vi "PSU_Output.vi"(8 "error in (no error)":errorcluster, 10 "Output %":dbl, 11 "DataCluster in":T1={"Core"={"Current VI Reference"=refnum, "Close Panel on Exit?"=FALSE, "Exit"=FALSE}, "Connections"={"cDAQ Therm"={"Task"="", "Connected"=FALSE, "Active"=FALSE}, "cDAQ Voltage"={"Task"="", "Connected"=FALSE, "Active"=FALSE}, "cDAQ ID"="", "Camera"={"Session"="", "Connected"=FALSE, "Active"=FALSE}, "PSU"={"Port"="", "Connected"=FALSE, "Active"=FALSE}}, "Data Acquisition"={"Setup"={"Label"="", "Operator"="", "Notes"="", "TempGrad"=1.0, "TargetTemp"=1.0, "Sample Volume"=1.0}, "Camera"={"Image"=refnum, "Save Image"=refnum, "Image Frequency"=20, "Rectangle"={"Left"=0, "Top"=0, "Right"=0, "Bottom"=0, "Rotation"=0.0}}, "Thermistor"={"Sample Size"=1, "Calibration"={"B0.100"=[], "R25"=[], "c"=[], "State"=[], "V_S"=5.0, "R_S"=100.0}, "Timing Mode"=14713}, "Partition"={"Data"=[], "Cell Label"="", "Cell Color"=0, "Height"=10, "Width"=16, "Grid"=[]}, "Queue"={"Queue"=refnum, "Size"=1}, "Sample Rate"=20, "Active"=FALSE, "Ready"=FALSE, "Graph Mode"=0}, "Control"={"Sample Rate"=1, "PID gains"={"proportional gain (Kc)"=1.0, "integral time (Ti, min)"=0.01, "derivative time (Td, min)"=0.0}}} {"Control"."PID gains"."derivative time (Td, min)" format="%.3f"; "Control"."PID gains"."integral time (Ti, min)" format="%.3f"; "Control"."PID gains"."proportional gain (Kc)" format="%.3f"; "Control"."Sample Rate" min=1 max=20 step=1 format="%.0f Samples/sec"; "Data Acquisition"."Graph Mode" items=["Average Temperature", "Individual Temperatures"]; "Data Acquisition"."Thermistor"."Timing Mode" items=["Automatic"=16097, "High Resolution"=10195, "High Speed"=14712, "Best 50 Hz Rejection"=14713, "Best 60 Hz Rejection"=14714, "Custom"=10137]; "Data Acquisition"."Thermistor"."Calibration"."R_S" min=0.1 max=1000.0 format="%#_g kOhm"; "Data Acquisition"."Thermistor"."Calibration"."V_S" min=5.0 max=48.0 format="%#_g V"; "Data Acquisition"."Thermistor"."Calibration"."R25" min=0.1 max=1000.0 format="%#_g kOhm"; "Data Acquisition"."Thermistor"."Calibration"."B0.100" min=100.0 max=10000.0 format="%#_g K"; "Data Acquisition"."Thermistor"."Sample Size" min=1 max=200; "Data Acquisition"."Sample Rate" min=20 max=240 format="%.0f samples/min"; "Data Acquisition"."Queue"."Size" min=1 max=200; "Data Acquisition"."Camera"."Rectangle"."Rotation" min=-90.0 max=90.0 step=1.0 format="%.2f"; "Data Acquisition"."Camera"."Rectangle"."Left" scale=0.0..1024.0; "Data Acquisition"."Camera"."Rectangle"."Right" scale=0.0..1024.0; "Data Acquisition"."Camera"."Image Frequency" min=1 max=60 step=1; "Data Acquisition"."Setup"."Sample Volume" min=0.0 max=500.0 format="%#_g µL"; "Data Acquisition"."Setup"."TargetTemp" min=-40.0 max=40.0 step=0.5 format="%#_g °C"; "Data Acquisition"."Setup"."TempGrad" min=-100.0 max=100.0 step=0.1 format="%#_g °C/min"}) -> (0 "error out":errorcluster, 1 "valid?":bool, 2 "Output % duplicate":dbl)   [LabVIEW 2020]
uses:
  DataCluster.ctl
  <vilib>/userDefined/High Color/IMAQdx.ctl
  <vilib>/vision/Image Controls.llb/IMAQ Image.ctl
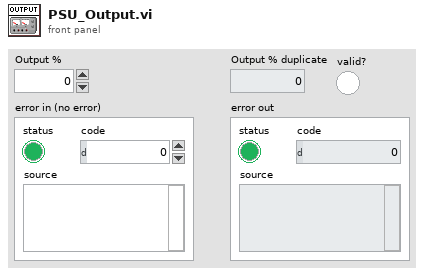
[diagram p1: front panel]
types:
  T1 = typedef "DataCluster.ctl" = cluster{"Core":cluster{"Current VI Reference":refnum<vi>, "Close Panel on Exit?":bool, "Exit":bool}, "Connections":cluster{"cDAQ Therm":cluster{"Task":refnum<k21>, "Connected":bool, "Active":bool}, "cDAQ Voltage":cluster{"Task":refnum<k21>, "Connected":bool, "Active":bool}, "cDAQ ID":string, "Camera":cluster{"Session":T2, "Connected":bool, "Active":bool}, "PSU":cluster{"Port":refnum<visa-resource-name>, "Connected":bool, "Active":bool}}, "Data Acquisition":cluster{"Setup":cluster{"Label":string, "Operator":string, "Notes":string, "TempGrad":dbl, "TargetTemp":dbl, "Sample Volume":dbl}, "Camera":cluster{"Image":T3, "Save Image":T3, "Image Frequency":i32, "Rectangle":T4}, "Thermistor":cluster{"Sample Size":i32, "Calibration":cluster{"B0.100":dbl[], "R25":dbl[], "c":dbl[][], "State":bool[], "V_S":dbl, "R_S":dbl}, "Timing Mode":i32}, "Partition":cluster{"Data":string[][], "Cell Label":string, "Cell Color":u32, "Height":i32, "Width":i32, "Grid":string[][]}, "Queue":cluster{"Queue":refnum<queue>, "Size":i32}, "Sample Rate":i32, "Active":bool, "Ready":bool, "Graph Mode":u16}, "Control":cluster{"Sample Rate":i32, "PID gains":cluster{"proportional gain (Kc)":dbl, "integral time (Ti, min)":dbl, "derivative time (Td, min)":dbl}}}
  T2 = typedef "IMAQdx.ctl" = refnum<k21>
  T3 = typedef "IMAQ Image.ctl" = refnum<image>
  T4 = typedef "IMAQ Rectangle" = cluster{"Left":i32, "Top":i32, "Right":i32, "Bottom":i32, "Rotation":dbl}
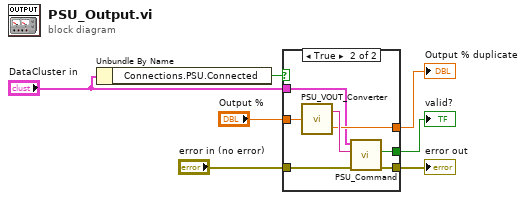
[diagram p0: block diagram]
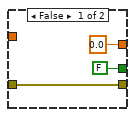
[diagram p2: hidden frame]
diagram:
  n1 = Unbundle By Name("DataCluster in") -> ("Connections.PSU.Connected"=w1:bool)
  n2 = case shown="True" w1 {
    tunnel: "Output %" -> [_ w16]
    tunnel: [0.0 ("Output % duplicate") w15] -> w6
    tunnel: "error in (no error)" -> [w8 w14]
    tunnel: [w8 w13] -> w4
    tunnel: "DataCluster in" -> [_ w12]
    tunnel: [FALSE ("valid?") w11] -> w3
    frame False {
    }
    frame True {
      n3 = call "PSU_VOUT_Converter.vi"("Output %"=w16) -> ("decimal integer string"=w17:string, "Output % duplicate"=w15:dbl)
      n4 = call "PSU_Command.vi"("error in (no error)"=w14, "command"=w17, "DataCluster"=w12) -> ("error out"=w13:errorcluster, "valid?"=w11:bool)  [unwired: 6 in, 1 out]
    }
  }
  "Output % duplicate" <- w6
  "error out" <- w4
  "valid?" <- w3
